vi "FlatToRichhwval_ExportRequest.vi"(5 "OutputClusterType":T1, 11 "InputCluster":T2) -> (3 "OutputCluster":T1)   [LabVIEW 2025, in "ExamplePluginOOBService_client.lvlib"]
uses:
  hwval_ExportRequest_Flat.ctl
  hwval_ExportRequest.ctl
  ExamplePluginOOBService_client.lvlib
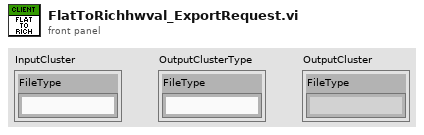
[diagram p1: front panel]
types:
  T1 = typedef "ExamplePluginOOBService_client.lvlib/hwval_ExportRequest.ctl" = cluster{"FileType":string}
  T2 = typedef "ExamplePluginOOBService_client.lvlib/hwval_ExportRequest_Flat.ctl" = cluster{"FileType":string}
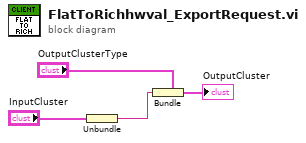
[diagram p0: block diagram]
diagram:
  n1 = Unbundle "Unbundle"("InputCluster") -> ("FileType"=w1:string)
  n2 = Bundle "Bundle"(cluster="OutputClusterType", "FileType"=w1) -> (→"OutputCluster":T1)
